vi "Core Actor - CLOSE - External Queues_Notifiers.vi"(8 "error in (no error)":errorcluster, 11 "Interface_Class in":refnum<class "Abstraction_Interface_Class.lvclass">) -> (0 "error out":errorcluster, 3 "Interface_Class out":refnum<class "Abstraction_Interface_Class.lvclass">)   [LabVIEW 2023, in "Abstraction_Interface.lvlib" / "Abstraction_Interface_Class.lvclass"]
uses:
  Abstraction_Interface_Class.lvclass
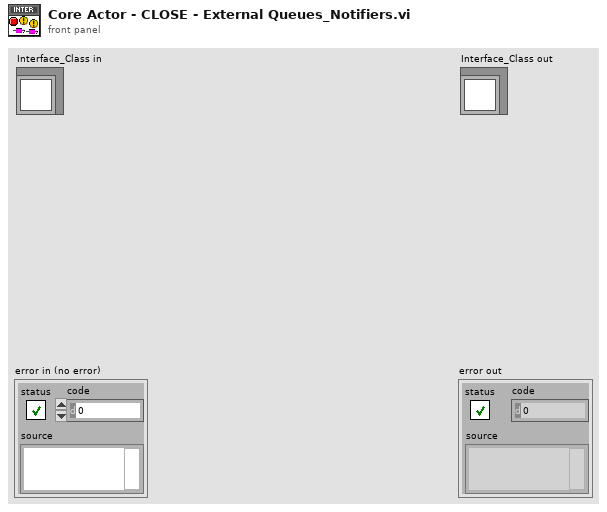
[diagram p1: front panel]
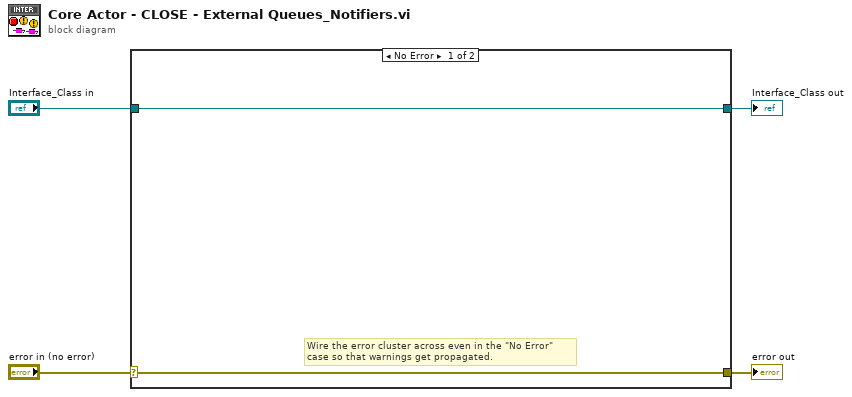
[diagram p0: block diagram]
diagram:
  n1 = case shown="No Error" "error in (no error)" {
    selector: "error in (no error)" -> [w5 w8]
    tunnel: [w5 w8] -> w3
    tunnel: [w6 w7] -> w1
    tunnel: "Interface_Class in" -> [w6 w7]
    frame No Error {
      # "Wire the error cluster across even in the \"No Error\"\ncase so that warnings get propagated."
    }
    frame Error {
    }
  }
  "error out" <- w3
  "Interface_Class out" <- w1
